vi "TDC_getHistogram.vi"(0 "Start Channel":i32, 5 "Stop Channel":i32, 7 "Reset":bool, 9 "Bin Count":i32, 11 "Error In":errorcluster) -> (1 "Data Count":i32, 2 "Data":i32[](array[numeric]), 3 "Exposure Time":i64, 4 "too Small":i32, 6 "too Large":i32, 8 "Starts":i32, 10 "Stops":i32, 15 "Error Out":errorcluster)   [LabVIEW 2011]
uses:
  tdcbase.dll
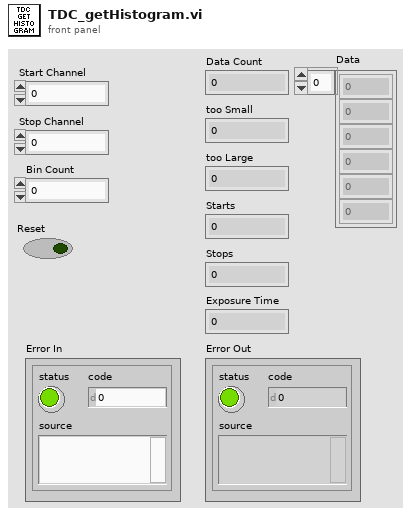
[diagram p1: front panel]
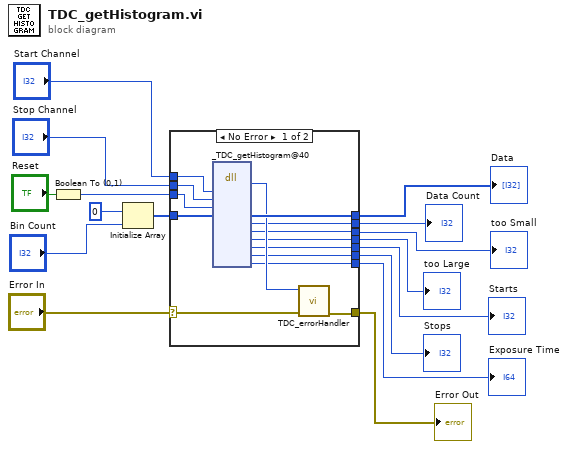
[diagram p0: block diagram]
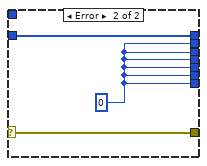
[diagram p2: hidden frame]
diagram:
  n1 = Boolean To (0,1)(Boolean="Reset") -> (0, 1=w12:i16)
  n2 = Initialize Array(0, "Bin Count") -> (w13:i32[])
  n3 = case shown="No Error" "Error In" {
    selector: "Error In" -> [w28 w33]
    tunnel: [w27 w33] -> w1
    tunnel: [w30 w32] -> w15
    tunnel: w13 -> [w29 w32]
    tunnel: w12 -> [w25 _]
    tunnel: [w22 w31] -> w11
    tunnel: "Stop Channel" -> [w24 _]
    tunnel: "Start Channel" -> [w23 _]
    tunnel: [w21 w31] -> w6
    tunnel: [w20 w31] -> w5
    tunnel: [w19 w31] -> w4
    tunnel: [w18 w31] -> w3
    tunnel: [w17 w31] -> w2
    frame No Error {
      n4 = dll-call lib="X:/tdcbase.dll" fn="_TDC_getHistogram@40"("ChStart"=w23, "chStop"=w24, "reset"=w25, "data"=w29) -> ("return type"=w26:i32, "data"=w30:i32[], "count"=w22:i32, "tooSmall"=w21:i32, "tooLarge"=w20:i32, "starts"=w19:i32, "stops"=w18:i32, "expTime"=w17:i64)  [unwired: 12 in, 2 out]
      n5 = call "TDC_errorHandler.vi"("Error In"=w28, "TDC Return Code"=w26) -> ("Error Out"=w27:errorcluster)  [unwired: 9 in]
    }
    frame Error {
      w31 = 0
    }
  }
  "Data" <- w15
  "Data Count" <- w11
  "too Small" <- w6
  "too Large" <- w5
  "Stops" <- w3
  "Exposure Time" <- w2
  "Starts" <- w4
  "Error Out" <- w1
